vi "Grid KeyDownCol.vi"(8 "error in (no error)":errorcluster caption="エラー入力（エラーなし）", 9 "VKey":T1, 10 "Char":i16, 11 "表関係クラスタ":T2) -> (0 "error out":errorcluster caption="エラー出力", 3 "破棄?":bool)   [LabVIEW 2014]
uses:
  <vilib>/event_ctls.llb/eventvkey.ctl
  Grid Parameter.ctl
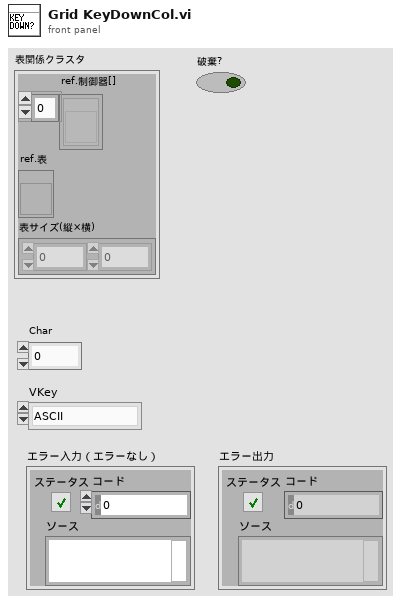
[diagram p1: front panel]
types:
  T1 = typedef "eventvkey.ctl" = enum16{"ASCII", "Enter", "Return", "Shift", "Ctrl", "Alt", "Cmd", "Opt", "Caps", "NumLock", "Clear", "Break", "Up", "Down", "Left", "Right", "Insert", "Delete", "Home", "End", "PageUp", "PageDown", "Escape", "Help", "Pause", "ScrollLock", "F1", "F2", "F3", "F4", "F5", "F6", "F7", "F8", "F9", "F10", "F11", "F12", "F13", "F14", "F15", "F16", "F17", "F18", "F19", "F20", "F21", "F22", "F23", "F24", "Play", "VolumeUp", "VolumeDown", "Mute", "Two Byte Char"}
  T2 = typedef "Grid Parameter.ctl" = cluster{"ref.制御器[]":refnum<vi>[], "ref.表":refnum<vi>, "表サイズ(縦×横)":i32[]}
  T3 = typedef "LVRowAndColumnTypeDef.ctl" = cluster{"Row":i32, "Column":i32}
  T4 = typedef "Clust ClassID.ctl" = enum16{"０", "１", "２", "３", "４", "５", "６", "色", "ブール", "９", "１０", "パス", "１２", "１３", "配列", "１５", "１６", "１７", "数値", "１９", "２０", "２１", "２２", "２３", "２４", "２５", "２６", "文字列", "２８", "２９", "３０", "３１", "３２", "３３", "リング", "Enum", "３６"}
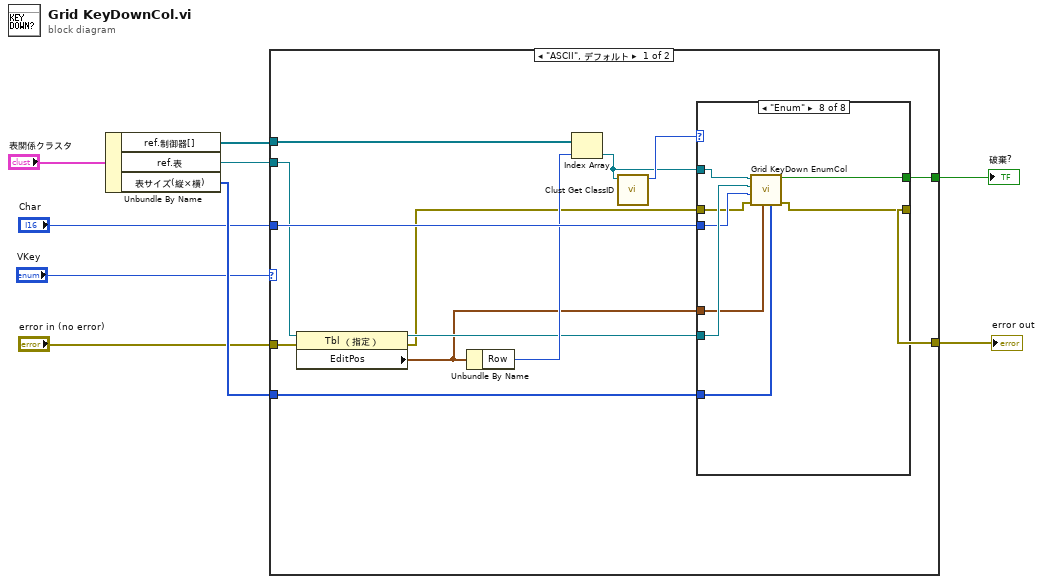
[diagram p0: block diagram]
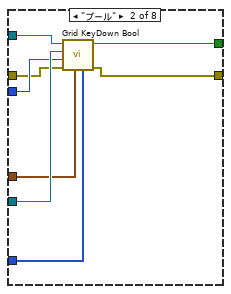
[diagram p3: hidden frame]
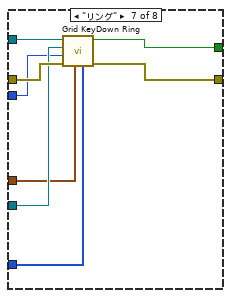
[diagram p8: hidden frame]
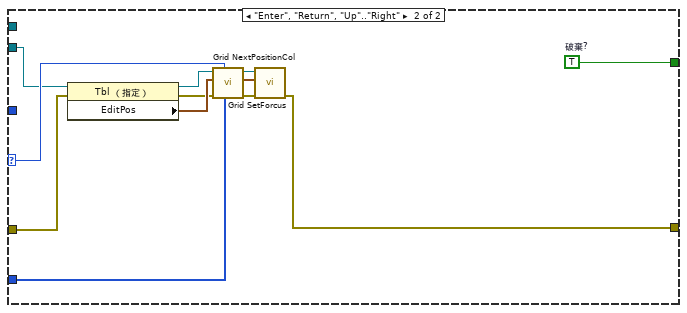
[diagram p9: hidden frame]
diagram:
  n1 = Unbundle By Name("表関係クラスタ") -> ("ref.制御器[]"=w8:refnum<vi>[], "ref.表"=w3:refnum<vi>, "表サイズ(縦×横)"=w9:i32[])
  n2 = case shown="\"ASCII\", デフォルト" "VKey" {
    selector: "VKey" -> [_ w58]
    tunnel: "Char" -> [w21 _]
    tunnel: [w22 w63] -> w4
    tunnel: w8 -> [w10 _]
    tunnel: w9 -> [w18 w62]
    tunnel: w3 -> [w16 w56]
    tunnel: "error in (no error)" -> [w13 w52]
    tunnel: [w12 w57] -> w1
    frame "ASCII", Default {
      n3 = property class="Tbl （指定）"(reference=w16, error in=w13) -> (reference out=w15:refnum<vi>, error out=w11:errorcluster, "EditPos"=w14:T3)
      n4 = Unbundle By Name(w14) -> ("Row"=w20:i32)
      n5 = Index Array(array=w10, index=w20) -> (element=w17:refnum<vi>)
      n6 = call "Clust Get ClassID.vi"("Ctl Refnum"=w17) -> ("ClassID"=w19:T4)  [unwired: 10 in]
      n7 = case shown="\"Enum\"" w19 {
        tunnel: w21 -> [_ w28 _ _ _ _ w39 w48]
        tunnel: w14 -> [_ w29 _ _ _ _ w38 w46]
        tunnel: [_ w27 _ _ _ _ w42 w51] -> w22
        tunnel: w17 -> [_ w31 _ _ _ _ w43 w50]
        tunnel: w18 -> [_ w26 _ _ _ _ w37 w45]
        tunnel: w15 -> [_ w30 _ _ _ _ w40 w49]
        tunnel: w11 -> [w23 w25 w32 w33 w34 w35 w41 w47]
        tunnel: [w23 w24 w32 w33 w34 w35 w36 w44] -> w12
        frame Default {
        }
        frame "ブール" {
          n8 = call "Grid KeyDown Bool.vi"("表サイズ(縦×横)"=w26, "EditPos"=w29, "error in (no error)"=w25, "Char"=w28, "ref.表"=w30, "Control入力"=w31) -> ("error out"=w24:errorcluster, "ブール"=w27:bool)  [unwired: 3 in, 1 out]
        }
        frame "パス" {
        }
        frame "配列" {
        }
        frame "数値" {
        }
        frame "文字列" {
        }
        frame "リング" {
          n9 = call "Grid KeyDown Ring.vi"("表サイズ(縦×横)"=w37, "EditPos"=w38, "エラー入力（エラーなし）"=w41, "Char"=w39, "ref.表"=w40, "Control入力"=w43) -> ("error out"=w36:errorcluster, "破棄?"=w42:bool)  [unwired: 3 in, 1 out]
        }
        frame "Enum" {
          n10 = call "Grid KeyDown EnumCol.vi"("表サイズ(縦×横)"=w45, "EditPos"=w46, "error in (no error)"=w47, "Char"=w48, "ref.表"=w49, "Control入力"=w50) -> ("error out"=w44:errorcluster, "ブール"=w51:bool)  [unwired: 3 in, 1 out]
        }
      }
    }
    frame "Enter", "Return", "Up".."Right" {
      w63 = TRUE  # 破棄?
      n11 = property class="Tbl （指定）"(reference=w56, error in=w52) -> (reference out=w53:refnum<vi>, error out=w54:errorcluster, "EditPos"=w55:T3)
      n12 = call "Grid NextPositionCol.vi"("表サイズ(縦x横)"=w62, "VKey(Right)"=w58, "error in (no error)"=w54, "EditPos入力"=w55, "ref.表"=w53) -> ("error out"=w60:errorcluster, "EditPos出力"=w59:T3, "ref.表(copy)"=w61:refnum<vi>)  [unwired: 4 in]
      n13 = call "Grid SetForcus.vi"("エラー入力（エラーなし）"=w60, "EditPos入力"=w59, "Table入力"=w61) -> ("error out"=w57:errorcluster)  [unwired: 6 in, 2 out]
    }
  }
  "破棄?" <- w4
  "error out" <- w1
